vi "GetCurrentPollCommandStatusFromCVT.vi"(8 "error in (no error)":errorcluster, 11 "Data Value Reference in":T1) -> (0 "error out":errorcluster, 2 "Command":T2, 3 "Data Value Reference out":T1)   [LabVIEW 2022 SP3, in "GIS Printer.lvclass"]
uses:
  GIS Printer.lvclass
  <vilib>/TELLC/Dynamic CVT API/TD Dynamic CVT DVR--ref.ctl
  Typedefs/PollCommandData-Cluster.ctl
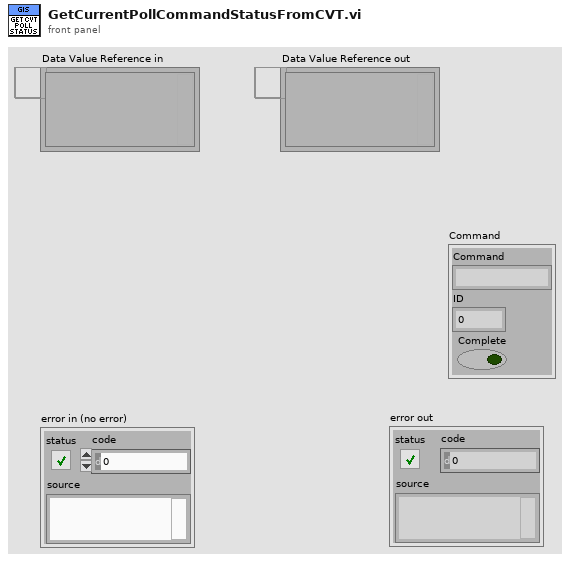
[diagram p1: front panel]
types:
  T1 = typedef "TD Dynamic CVT DVR--ref.ctl" = refnum<data-value>
  T2 = typedef "PollCommandData-Cluster.ctl" = cluster{"Command":string, "ID":i32, "Complete":bool}
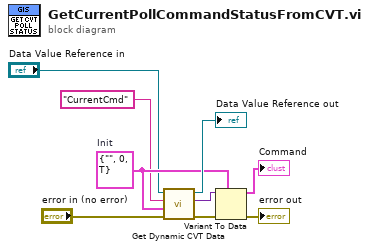
[diagram p0: block diagram]
diagram:
  w6 = T2 {"Command"="", "ID"=0, "Complete"=TRUE}  # Init
  n1 = call <vilib>:"Get Dynamic CVT Data.vi"("error in (no error)"="error in (no error)", "default value (empty variant)"=w6, "DataName"="CurrentCmd", "dCVT DVR"="Data Value Reference in") -> ("error out"=w7:errorcluster, "value"=w5:variant, "dCVT DVR out"=→"Data Value Reference out":T1)  [unwired: 4 in, 1 out]
  n2 = Variant To Data(error in=w7, type=w6, Variant=w5) -> (data=→"Command":T2, error out=→"error out":errorcluster)
